vi "Finish.vi"   [LabVIEW 2017]
doc: "This VI is called just before exiting. It is expected to close I/O refnum, save collected data, etc."
uses:
  <vilib>/Rock Robotics/WPI/Utilities/WPI_GetSetVariantRefNum.vi
types:
  T1 = typedef "WPI_RelayDevRef.ctl" = cluster{"DevStatus":errorcluster, "Relay Channel":T2, "Relay Direction":T3}
  T2 = typedef "FPGA_DIORelayChannel.ctl" = enum8{"Relay 0", "Relay 1", "Relay 2", "Relay 3", "Invalid"}
  T3 = typedef "WPI_RelayDirection.ctl" = enum16{"Both directions", "Forward only", "Reverse only"}
  T4 = typedef "WPI_CompressorDevRef.ctl" = cluster{"DevStatus":errorcluster, "Pneumatics Control Module":u8}
  T5 = typedef "WPI_RobotDriveDevRef.ctl" = cluster{"DevStatus":errorcluster, "Motors[]":T6[], "Square Inputs":bool, "Max Output":dbl}
  T6 = typedef "WPI_MotorControlDeviceRef.ctl" = cluster{"DeviceStatus":errorcluster, "Type":T7, "PWM":cluster{"PWM Channel":T8, "DeadBand":T9}, "CAN":cluster{"Device Number":u8, "SetOutput VI Ref":variant, "GetOutput VI Ref":variant, "Enable VI Ref":variant, "Disable VI Ref":variant, "Data":variant}, "Invert":bool, "DIO PWM":cluster{"PWM \"Enable\" Channel":T8, "DIOChannel":T10, "PWM Rate":dbl}}
  T7 = typedef "WPI_MotorControlType.ctl" = enum16{"PWM", "CAN", "DIO PWM"}
  T8 = typedef "FPGA_DIOPWMChannel.ctl" = enum8{"PWM 0", "PWM 1", "PWM 2", "PWM 3", "PWM 4", "PWM 5", "PWM 6", "PWM 7", "PWM 8", "PWM 9", "PWM MXP 0", "PWM MXP 1", "PWM MXP 2", "PWM MXP 3", "PWM MXP 4", "PWM MXP 5", "PWM MXP 6", "PWM MXP 7", "PWM MXP 8", "PWM MXP 9", "Invalid"}
  T9 = typedef "WPI_PWMDeadband.ctl" = cluster{"Name":string, "maxPositivePwm":i32, "minPositivePwm":i32, "centerPwm":i32, "maxNegativePwm":i32, "minNegativePwm":i32, "angularRange":u16}
  T10 = typedef "FPGA_DIOChannel.ctl" = enum8{"DIO 0", "DIO 1", "DIO 2", "DIO 3", "DIO 4", "DIO 5", "DIO 6", "DIO 7", "DIO 8", "DIO 9", "DIO MXP 0", "DIO MXP 1", "DIO MXP 2", "DIO MXP 3", "DIO MXP 4", "DIO MXP 5", "DIO MXP 6", "DIO MXP 7", "DIO MXP 8", "DIO MXP 9", "DIO MXP 10", "DIO MXP 11", "DIO MXP 12", "DIO MXP 13", "DIO MXP 14", "DIO MXP 15", "SPI Port CS1", "SPI Port CS2", "SPI Port CS3", "SPI Port MISO", "SPI Port MOSI", "Invalid"}
  T11 = typedef "WPI_JoystickDevRef.ctl" = cluster{"Device":T12}
  T12 = typedef "WPI_JoystickDeviceEnum.ctl" = enum16{"USB 0", "USB 1", "USB 2", "USB 3", "USB 4", "USB 5"}
  T13 = typedef "WPI_SwitchDevRef.ctl" = cluster{"DevStatus":errorcluster, "DIO Channel":T10, "CntIndex":T14, "Normally Closed":bool}
  T14 = typedef "FPGA_CounterCtrSystemIndex.ctl" = enum8{"Ctr 0", "Ctr 1", "Ctr 2", "Ctr 3", "Ctr 4", "Ctr 5", "Ctr 6", "Ctr 7", "Invalid"}
  T15 = typedef "WPI_SolenoidDevRef.ctl" = cluster{"DevStatus":errorcluster, "Pneumatics Control Module":u8, "Forward Solenoid Channel":T16, "Reverse Solenoid Channel":T16}
  T16 = typedef "WPI_SolenoidChannel.ctl" = enum8{"Solenoid 0", "Solenoid 1", "Solenoid 2", "Solenoid 3", "Solenoid 4", "Solenoid 5", "Solenoid 6", "Solenoid 7", "Invalid"}
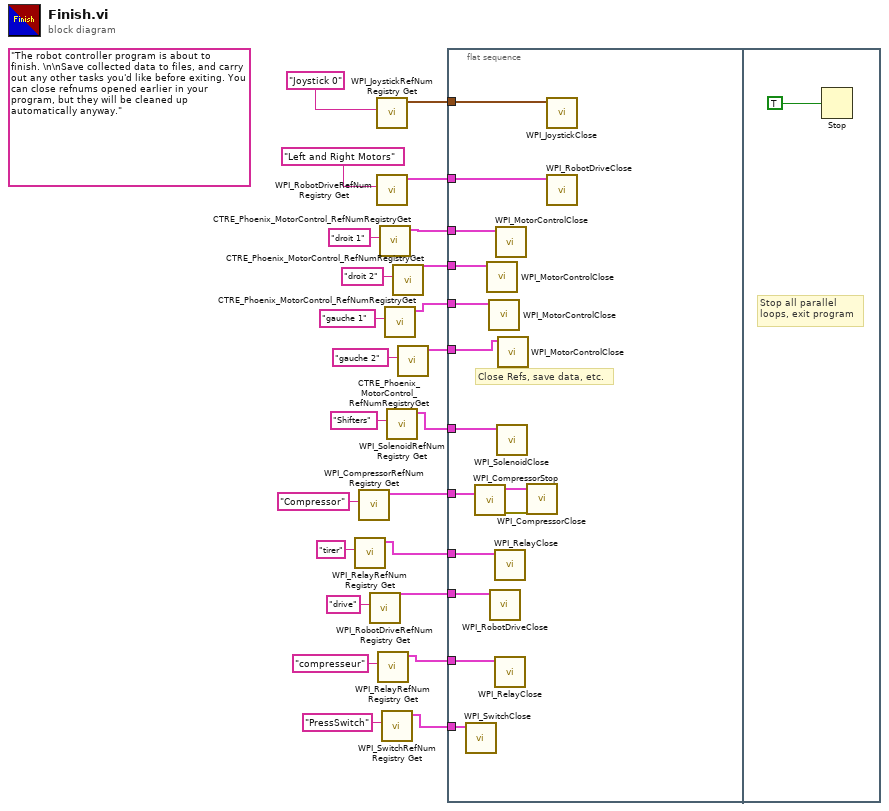
[diagram p0: block diagram]
diagram:
  (unwired) "The robot controller program is about to finish. \n\nSave collected data to files, and carry out any other tasks you'd like before exiting. You can close refnums opened earlier in your program, but they will be cleaned up automatically anyway."
  n1 = call <vilib>:"WPI_RelayRefNum Registry Get.vi"("refnum name"="tirer") -> ("RelayDevRef"=w7:T1)  [unwired: 9 in, 1 out]
  n2 = call <vilib>:"WPI_CompressorRefNum Registry Get.vi"("refnum name"="Compressor") -> ("CompressorDevRef"=w10:T4)  [unwired: 9 in, 1 out]
  n3 = call <vilib>:"WPI_RobotDriveRefNum Registry Get.vi"("refnum name"="drive") -> ("RobotDriveDevRef"=w5:T5)  [unwired: 9 in, 1 out]
  n4 = call <vilib>:"WPI_JoystickRefNum Registry Get.vi"("refnum name"="Joystick 0") -> ("JoystickDevRef"=w21:T11)  [unwired: 1 in, 9 out]
  n5 = call <vilib>:"WPI_RobotDriveRefNum Registry Get.vi"("refnum name"="Left and Right Motors") -> ("RobotDriveDevRef"=w22:T5)  [unwired: 1 in, 9 out]
  n6 = call <vilib>:"WPI_RelayRefNum Registry Get.vi"("refnum name"="compresseur") -> ("RelayDevRef"=w3:T1)  [unwired: 9 in, 1 out]
  n7 = call "CTRE_Phoenix_MotorControl_RefNumRegistryGet.vi"("refnum name"="droit 1") -> ("PhoenixMotorControlDevRef"=w16:T6)  [unwired: 9 in, 1 out]
  n8 = call <vilib>:"WPI_SwitchRefNum Registry Get.vi"("refnum name"="PressSwitch") -> ("SwitchDevRef"=w1:T13)  [unwired: 9 in, 1 out]
  n9 = call "CTRE_Phoenix_MotorControl_RefNumRegistryGet.vi"("refnum name"="gauche 1") -> ("PhoenixMotorControlDevRef"=w14:T6)  [unwired: 9 in, 1 out]
  n10 = call <vilib>:"WPI_SolenoidRefNum Registry Get.vi"("refnum name"="Shifters") -> ("SolenoidDevRef"=w12:T15)  [unwired: 9 in, 1 out]
  n11 = call "CTRE_Phoenix_MotorControl_RefNumRegistryGet.vi"("refnum name"="droit 2") -> ("PhoenixMotorControlDevRef"=w15:T6)  [unwired: 9 in, 1 out]
  n12 = call "CTRE_Phoenix_MotorControl_RefNumRegistryGet.vi"("refnum name"="gauche 2") -> ("PhoenixMotorControlDevRef"=w13:T6)  [unwired: 9 in, 1 out]
  n13 = flat-sequence {
    tunnel: w22 -> [w38]
    tunnel: w21 -> [w37]
    tunnel: w16 -> [w36]
    tunnel: w15 -> [w35]
    tunnel: w14 -> [w34]
    tunnel: w13 -> [w33]
    tunnel: w12 -> [w32]
    tunnel: w10 -> [w29]
    tunnel: w7 -> [w28]
    tunnel: w5 -> [w27]
    tunnel: w3 -> [w26]
    tunnel: w1 -> [w25]
    frame #0 {
      # "Close Refs, save data, etc."
      n14 = call <vilib>:"WPI_SwitchClose.vi"("SwitchDevRef"=w25) -> ()  [unwired: 10 in, 1 out]
      n15 = call <vilib>:"WPI_CompressorStop.vi"("CompressorDevRef"=w29) -> ("error out"=w31:errorcluster, "CompressorDevRef"=w30:T4)  [unwired: 9 in]
      n16 = call <vilib>:"WPI_MotorControlClose.vi"("MotorControlDevRef"=w35) -> ()  [unwired: 10 in, 1 out]
      n17 = call <vilib>:"WPI_MotorControlClose.vi"("MotorControlDevRef"=w34) -> ()  [unwired: 10 in, 1 out]
      n18 = call <vilib>:"WPI_RobotDriveClose.vi"("RobotDriveDevRef"=w27) -> ()  [unwired: 10 in, 1 out]
      n19 = call <vilib>:"WPI_RelayClose.vi"("RelayDevRef"=w28) -> ()  [unwired: 10 in, 1 out]
      n20 = call <vilib>:"WPI_RelayClose.vi"("RelayDevRef"=w26) -> ()  [unwired: 10 in, 1 out]
      n21 = call <vilib>:"WPI_MotorControlClose.vi"("MotorControlDevRef"=w36) -> ()  [unwired: 10 in, 1 out]
      n22 = call <vilib>:"WPI_SolenoidClose.vi"("SolenoidDevRef"=w32) -> ()  [unwired: 10 in, 1 out]
      n23 = call <vilib>:"WPI_MotorControlClose.vi"("MotorControlDevRef"=w33) -> ()  [unwired: 10 in, 1 out]
      n24 = call <vilib>:"WPI_CompressorClose.vi"("error in (no error)"=w31, "CompressorDevRef"=w30) -> ()  [unwired: 9 in, 1 out]
      n25 = call <vilib>:"WPI_JoystickClose.vi"("JoystickDevRef"=w37) -> ()  [unwired: 11 out]
      n26 = call <vilib>:"WPI_RobotDriveClose.vi"("RobotDriveDevRef"=w38) -> ()  [unwired: 1 in, 10 out]
    }
    frame #1 {
      # "Stop all parallel\nloops, exit program"
      n27 = Stop(stop? (T)=TRUE ("Quit")) -> ()
    }
  }
